vi "Lock Publication.vi"(4 "Return Error Transport":refnum<class "ITransport.lvclass">, 6 "Publisher ID":string, 7 "PublicationPolicy":refnum<class "IPublicationPolicy.lvclass">, 8 "error in (no error)":errorcluster, 9 "Datum Type":variant, 10 "Datum Name":string, 11 "IMediator In":refnum<class "IMediator.lvclass">) -> (0 "error out":errorcluster, 3 "IMediator Out":refnum<class "IMediator.lvclass">)   [LabVIEW 2018, in "MVA Framework.lvlib" / "IMediator.lvlib" / "IMediator.lvclass"]
doc: "抽象方法\n锁定发布者"
uses:
  IMediator.lvclass
  composed-transport/Source/ITransport/ITransport.lvclass
  IPublicationPolicy/IPublicationPolicy.lvclass
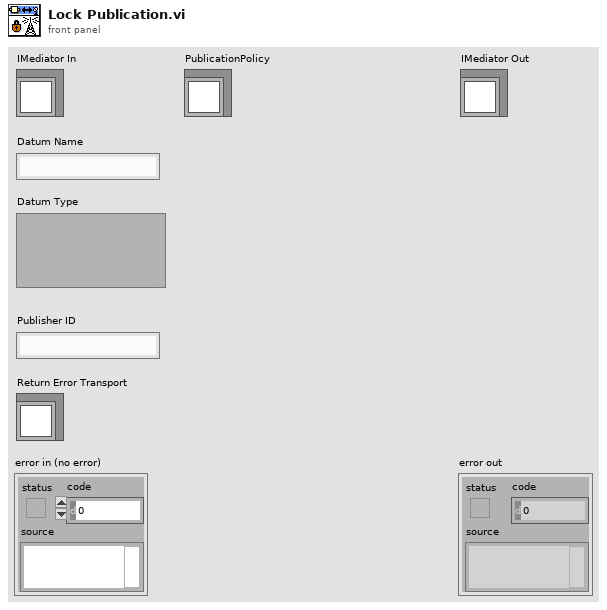
[diagram p1: front panel]
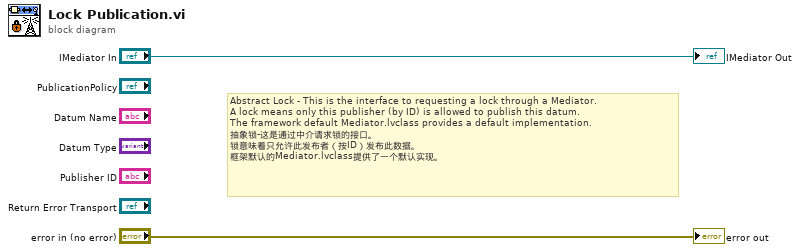
[diagram p0: block diagram]
diagram:
  # "Abstract Lock - This is the interface to requesting a lock through a Mediator.\nA lock means only this publisher (by ID) is allowed to publish this datum.\nThe framework default Mediator.lvclass provides a default implementation.\n抽象锁-这是通过中介请求锁的接口。\n锁意味着只允许此发布者（按ID）发布此数据。\n框架默认的Mediator.lvclass提供了一个默认实现。"
  "error out" <- "error in (no error)"
  "IMediator Out" <- "IMediator In"
